vi "Ideal Sub Layout.vi"() -> ()   [LabVIEW 2018]
uses:
  support/mqtt/Controls/Connect_Flags.ctl
  support/mqtt/Controls/QoS.ctl
  support/mqtt/MQTT_Functions.lvlib
panel:
  in  "Frequency  2":dbl
  out "Log output":bool
  in  "String":string
  in  "Remove":bool
  out "Logging":bool
  in  "Frequency":dbl
  out "Live View":string
  in  "Add All":bool
  in  "List of All Subscribed Topics":i32(listbox)
  in  "Subscribe":bool
  in  "Add":bool
  out "Separate VI Window":bool
  in  "stop":bool
  in  "MQTT Code":string
  in  "Subscriber Topics":string(combo)
  in  "port":u16=1883
  in  "Client ID":string="subcriber"
  in  "Connect Flags":T1={"user name"=FALSE, "password"=FALSE, "will retain"=FALSE, "will flag"=FALSE, "clean session"=TRUE, "reserved"=FALSE, "will QoS"=enum."At most once"}
  in  "Ip Address":string
  in  "Connect":bool
  # "This is the Area which is mostly the MQTT library imported. \nnot sure what will be used, but typically Clean session each time no PW or UN"
  # "This Area will be where the MQTT Topics are selected.\n* Combo box populated from .ini file will show all topics that can be selected\n*MQTT code box shows the subscribe code to be sent to double check\n*List Box will have all the Topics that are added to be  subsciber - when you press \"Add\" they appear in here\n*Live view is if the user has not selected \"Separate VI Window\" and wants to see all subscribe message responses \nalternating  by the \"Frequency\"\n*Logging is to take the raw String test and log to file from \"Live view\""
  # "This Area has controls for teh topics and when to subscribe\n*\"Separate VI Window\" when selected all the List of subscribed topics in the list box \nopen in a seporate Window all running and all have Frequency controls \n*\"add\" adds the selected \"subscriber topic\" from the combo box to the \"List of subscribed topics\" list box\n* \"Add All\" selects all the topics in the \"Subscriber Topics\" combo Box to the   \"List of subscribed topics\" list box\n*Subscribe - then Sets the list and starts getting back responses. \nif more want to be added, you select \"Stop\" Add or Remove, then subscribe again \n*\"remove\" removes teh selected topic highlighted in the \"Subscriber Topics\" Combo box, from the \"list of All \nsubscribe topics\""
  # "Pop out VI General Look"
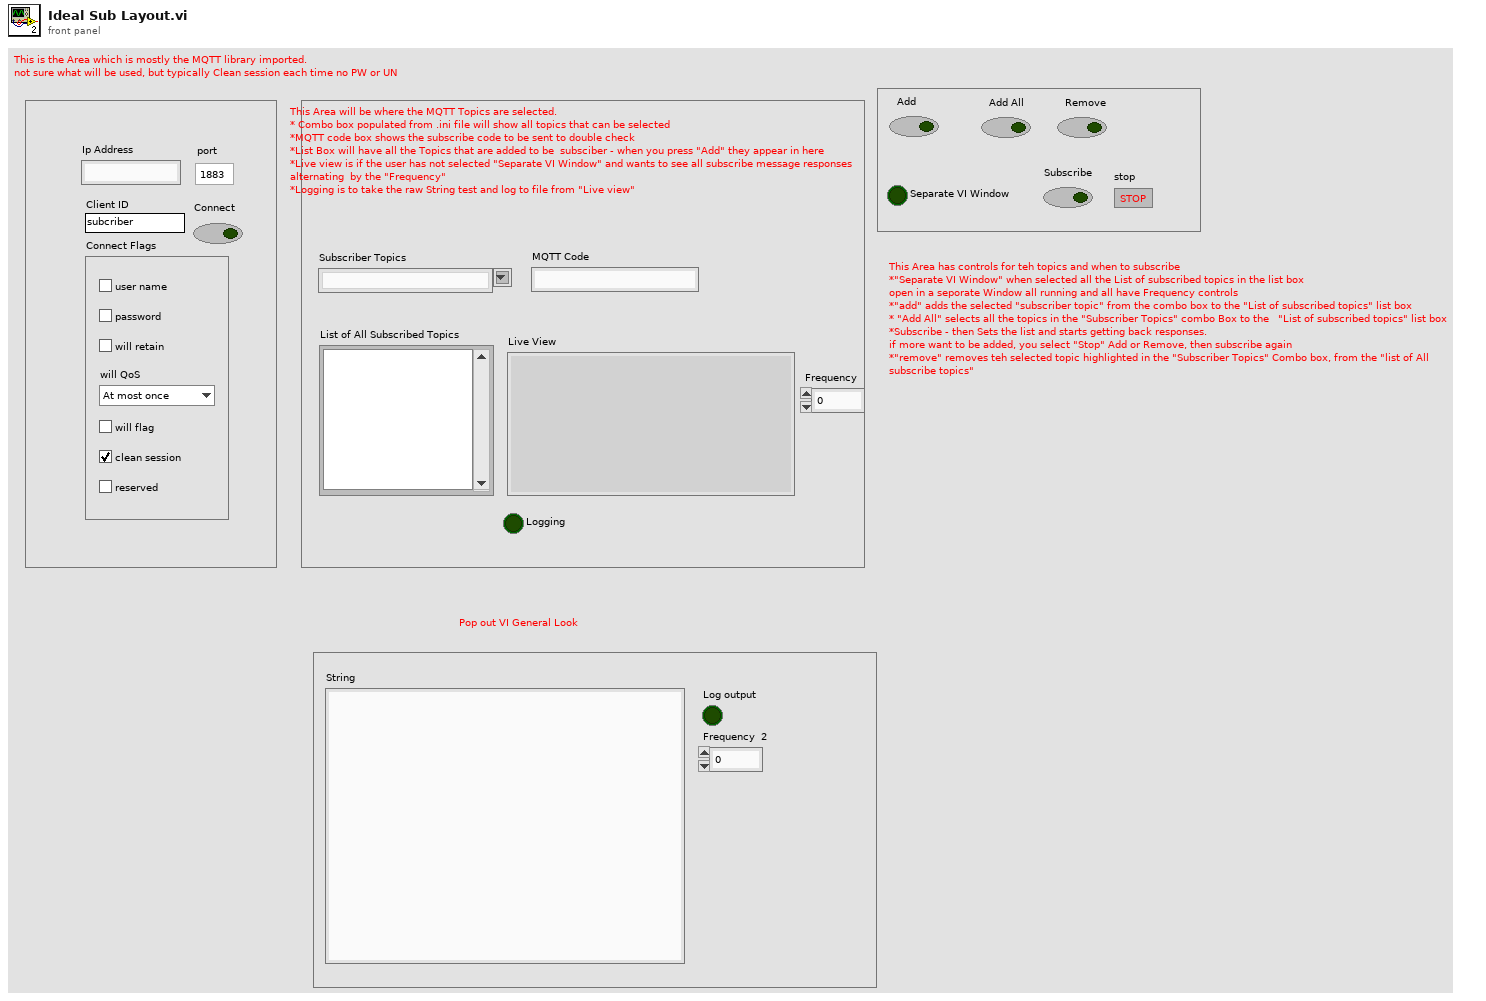
[diagram p1: front panel]
types:
  T1 = typedef "MQTT_Functions.lvlib/Connect_Flags.ctl" = cluster{"user name":bool, "password":bool, "will retain":bool, "will flag":bool, "clean session":bool, "reserved":bool, "will QoS":T2}
  T2 = typedef "MQTT_Functions.lvlib/QoS.ctl" = enum8{"At most once", "At least once", "Exactly once", "Reserved"}
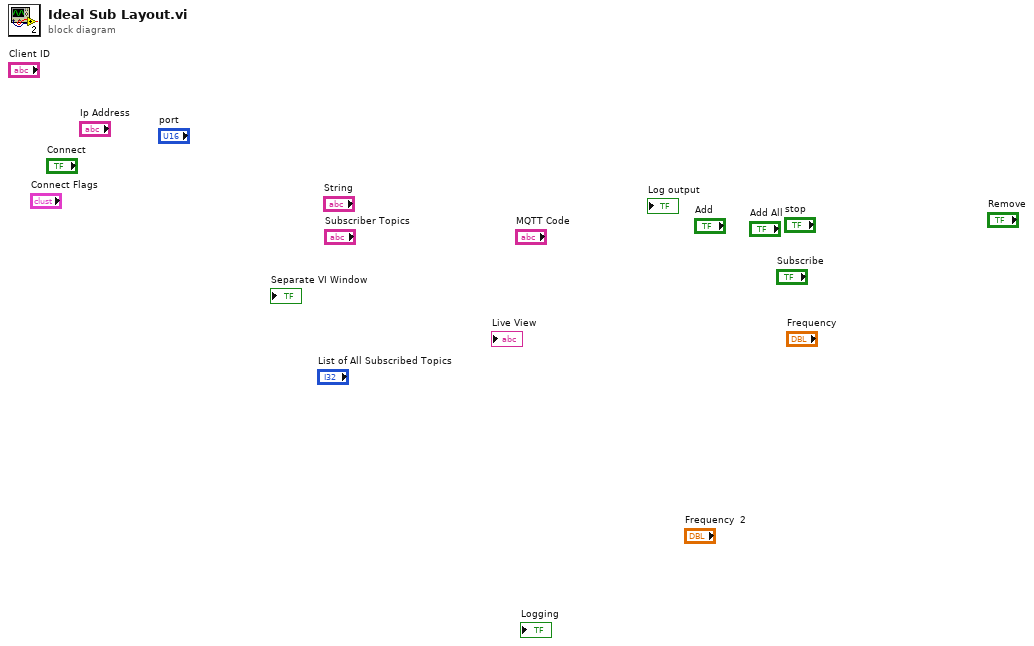
[diagram p0: block diagram]
diagram:
